vi "Ignore_Channel_evaluate.vi"(4 "Column Index":i32, 5 "Ignore When String":string, 6 "Template Names":string[](array[string]), 7 "Data":string[][](array[string])) -> (3 "Data Out":string[][](array[string]))   [LabVIEW 2018]
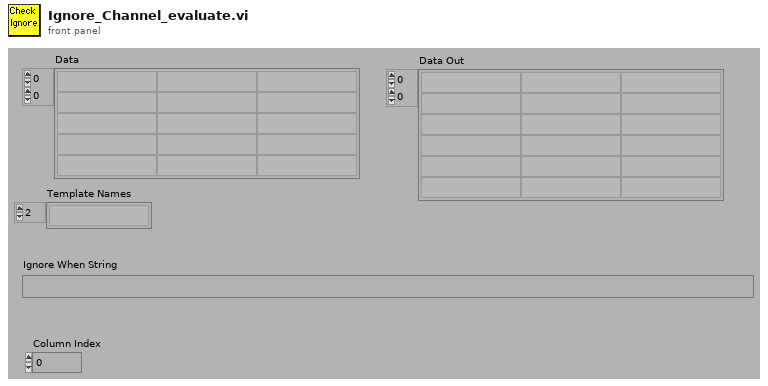
[diagram p1: front panel]
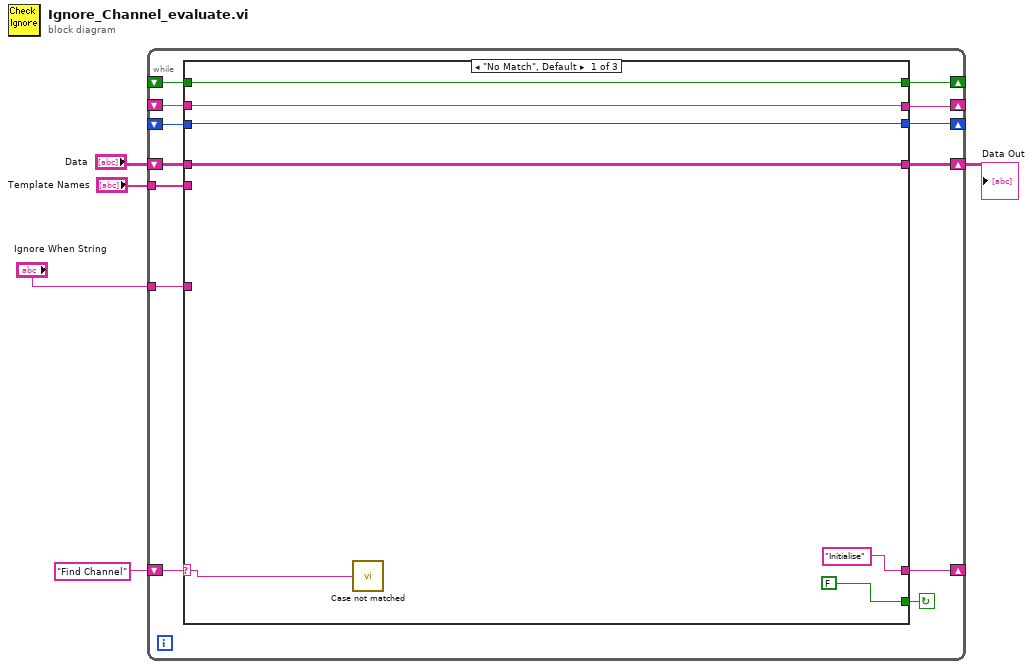
[diagram p0: block diagram]
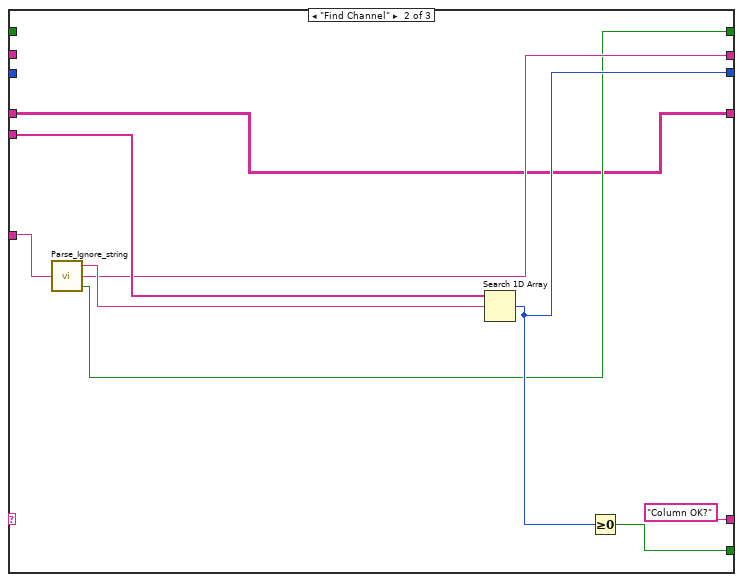
[diagram p2: hidden frame]
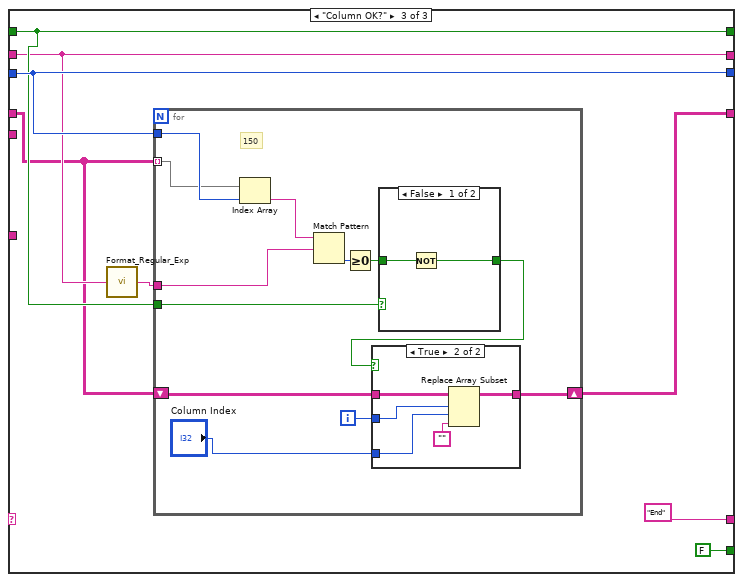
[diagram p3: hidden frame]
diagram:
  n1 = while {
    shift-left: _ -> [w13]
    shift-right: [w14] -> _
    tunnel: "Template Names" -> [w15]
    shift-left: "Find Channel" -> [w16]
    shift-right: [w17] -> _
    tunnel: "Ignore When String" -> [w12]
    shift-right: [w11] -> _
    shift-left: _ -> [w10]
    shift-right: [w9] -> _
    shift-left: _ -> [w8]
    shift-right: [w7] -> w1
    shift-left: "Data" -> [w6]
    stop <- w18 continue-if-true
    n2 = case shown="\"No Match\", Default" w16 {
      selector: w16 -> [w19 _ _]
      tunnel: [FALSE w31 FALSE] -> w18
      tunnel: ["Initialise" "Column OK?" "End"] -> w17
      tunnel: w15 -> [_ w33 _]
      tunnel: [w23 w32 w40] -> w14
      tunnel: w13 -> [w23 _ w40]
      tunnel: w12 -> [_ w27 _]
      tunnel: [w21 w29 w37] -> w11
      tunnel: w10 -> [w21 _ w37]
      tunnel: [w22 w28 w38] -> w9
      tunnel: w8 -> [w22 _ w38]
      tunnel: [w20 w26 w35] -> w7
      tunnel: w6 -> [w20 w26 w36]
      frame "No Match", Default {
        n3 = call "Case not matched.vi"("Case Name not Matched"=w19) -> ()
      }
      frame "Find Channel" {
        n4 = call "Parse_Ignore_string.vi"("Ignore When String"=w27) -> ("Channel Name"=w30:string, "Search String"=w29:string, "Does Contain"=w28:bool)
        n5 = Search 1D Array(1D array=w33, element=w30) -> (index of element=w32:i32)  [unwired: 1 out]
        n6 = Greater Or Equal To 0?(x=w32) -> (x >= 0?=w31:bool)
      }
      frame "Column OK?" {
        n7 = call "Format_Regular_Exp.vi"("Regular expression"=w37) -> ("Case Insensitive for html"=w41:string)
        n8 = for {
          tunnel: w36 -> [w51] mode=indexing
          tunnel: w40 -> [w52]
          tunnel: w41 -> [w54]
          tunnel: w38 -> [w53]
          shift-right: [w43] -> w35
          shift-left: w36 -> [w44]
          i -> [w47]
          # "150"
          n9 = Index Array(array=w51, index=w52) -> (element=w50:string)
          n10 = Match Pattern(string=w50, regular expression=w54) -> (offset past match=w49:i32)  [unwired: 4 out]
          n11 = Greater Or Equal To 0?(x=w49) -> (x >= 0?=w48:bool)
          n12 = case shown="False" w53 {
            tunnel: [w61 w63] -> w45
            tunnel: w48 -> [w62 w63]
            frame False {
              n13 = Not(x=w62) -> (.not. x?=w61:bool)
            }
            frame True {
            }
          }
          n14 = case shown="True" w45 {
            tunnel: w44 -> [w55 w60]
            tunnel: w47 -> [_ w57]
            tunnel: [w55 w59] -> w43
            tunnel: "Column Index" -> [_ w56]
            frame False {
            }
            frame True {
              n15 = Replace Array Subset(array=w60, new element="", index (row)=w57, index (col)=w56) -> (w59:string[][])
            }
          }
        }
      }
    }
  }
  "Data Out" <- w1
